vi "checkGST.vi"(0 "reference in":refnum<class "excelFile.lvclass">, 2 "TSR_details":T1={"Company/Institution:"="", "Address:"="", "Department:"="", "City:"="", "Post Code:"="", "Country:"="", "Contact:"="", "Ref:"="", "Issue description:"="", "Actions:"="", "TYPE:"="Repair", "Shipping:"=0, "Discount:"=0, "dataIN"=[], "Device type:"="microQuark", "Serial Number:"="", "PMC number:"="", "Labour Hours:"=0.0, "Service Location:"=FALSE, "start_hour"="", "end_hour"="", "o2_exp_date"="", "GST"=TRUE}, 5 "error in (no error)":errorcluster) -> (14 "reference out":refnum<class "excelFile.lvclass">, 19 "error out":errorcluster)   [LabVIEW 2016, in "excelFile.lvclass"]
uses:
  excelFile.lvclass
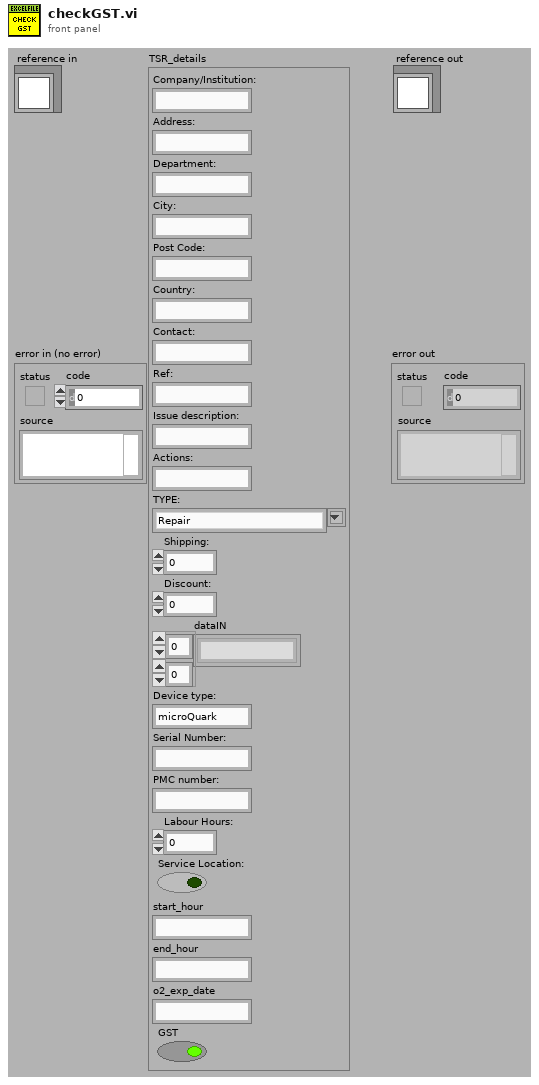
[diagram p1: front panel]
types:
  T1 = cluster{"Company/Institution:":string, "Address:":string, "Department:":string, "City:":string, "Post Code:":string, "Country:":string, "Contact:":string, "Ref:":string, "Issue description:":string, "Actions:":string, "TYPE:":string, "Shipping:":i32, "Discount:":i32, "dataIN":string[][], "Device type:":string, "Serial Number:":string, "PMC number:":string, "Labour Hours:":dbl, "Service Location:":bool, "start_hour":string, "end_hour":string, "o2_exp_date":string, "GST":bool}
  T2 = typedef "excelFile.lvclass/ObjectAttributesRef.ctl" = refnum<data-value>
  T3 = typedef "excelFile.lvclass/ObjectAttributes.ctl" = cluster{"MyAttribute":dbl, "path":string, "Refnum Excel":cluster{"Excel._Application":refnum<k7>, "Workbooks":refnum<k7>, "Open":refnum<k7>}, "data":string[][][], "save":bool, "fileType":T4, "rowsColor":u32[], "python_ref":refnum<class "python.lvclass">, "items_rows":i32[], "excel_range":i32[][], "TSR":cluster{"number":string, "TSR_path":path, "service_path":path, "email_to":string}, "excel_already_opened?":bool, "file_already_opened?":bool, "excel_protected_opened?":bool, "Refnum Cluster Worksheets":cluster{"Excel._Application":refnum<k7>, "Workbooks":refnum<k7>, "Open":refnum<k7>, "Worksheets":refnum<k7>, "Excel._Worksheet":refnum<k7>}, "#_rows_defective":i32, "#_rows_spare":i32}
  T4 = typedef "excelFile.lvclass/fileType.ctl" = enum16{"devices", "items", "partsTracking", "TSR"}
  T5 = cluster{"Excel._Application":refnum<k7>, "Workbooks":refnum<k7>, "Open":refnum<k7>, "Worksheets":refnum<k7>, "Excel._Worksheet":refnum<k7>}
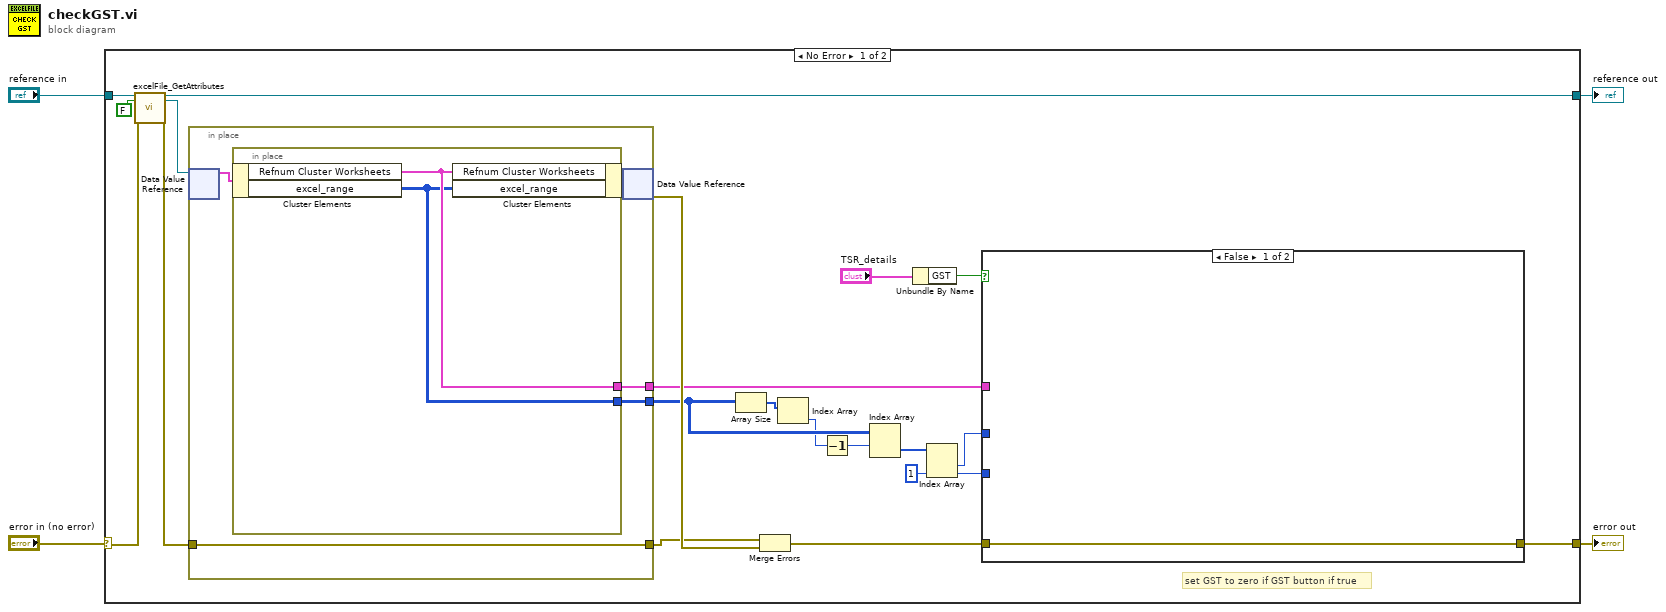
[diagram p0: block diagram]
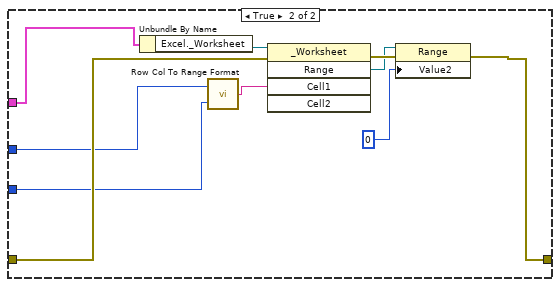
[diagram p2: hidden frame]
diagram:
  n1 = case shown="No Error" "error in (no error)" {
    selector: "error in (no error)" -> [w22 w45]
    tunnel: [w15 w45] -> w3
    tunnel: [w20 w44] -> w1
    tunnel: "reference in" -> [w24 w44]
    frame No Error {
      # "set GST to zero if GST button if true"
      n2 = call "excelFile_GetAttributes.vi"("reference in"=w24, "return data? (T)"=FALSE, "error in (no error)"=w22) -> ("reference out"=w20:refnum<class "excelFile.lvclass">, "attributes ref"=w19:T2, "error out"=w21:errorcluster)  [unwired: 13 in, 1 out]
      n3 = in-place {
        in-place-border: w21 -> [w39]
        in-place-border: [w39] -> w17
        in-place-border: [w38] -> w16
        in-place-border: [w37] -> w13
        n4 = in-place-dvr #1(w19) -> (w40:T3)  [unwired: 1 out]
        n5 = in-place {
          in-place-border: [w43] -> w38
          in-place-border: [w42] -> w37
          n6 = in-place-cluster #2(w40) -> ("Refnum Cluster Worksheets"=w43:T5, "excel_range"=w42:i32[][])
          n7 = in-place-cluster #2("Refnum Cluster Worksheets"=w43, "excel_range"=w42) -> (w41:T3)
        }
        n8 = in-place-dvr #1(w41) -> (w25:errorcluster)  [unwired: 1 out]
      }
      n9 = Array Size(array=w13) -> (size(s)=w12:i32[])
      n10 = Merge Errors(w17, w25) -> (w18:errorcluster)
      n11 = Index Array(array=w12) -> (element=w11:i32)  [unwired: 1 in]
      n12 = Decrement(x=w11) -> (x-1=w5:i32)
      n13 = Index Array(array=w13, index (row)=w5) -> (element=w10:i32[])  [unwired: 1 in]
      n14 = Unbundle By Name("TSR_details") -> ("GST"=w6:bool)
      n15 = Index Array(array=w10, index #2=1 ("index")) -> (element #1=w9:i32, element #2=w8:i32)  [unwired: 1 in]
      n16 = case shown="False" w6 {
        tunnel: w18 -> [w26 w36]
        tunnel: w16 -> [_ w35]
        tunnel: [w26 w34] -> w15
        tunnel: w9 -> [_ w29]
        tunnel: w8 -> [_ w28]
        frame False {
        }
        frame True {
          n17 = Unbundle By Name(w35) -> ("Excel._Worksheet"=w30:refnum<k7>)
          n18 = call <userlib>:"Row Col To Range Format.vi"("Column"=w28, "Row"=w29) -> ("Output String"=w33:string)
          n19 = invoke class="_Worksheet" method="Range"(reference=w30, error in=w36, "Cell1"=w33) -> (error out=w32:errorcluster, "Range"=w31:refnum<k7>)  [unwired: 2 in, 3 out]
          n20 = property class="Range"(reference=w31, error in=w32, "Value2"=0 ("index")) -> (error out=w34:errorcluster)  [unwired: 1 out]
        }
      }
    }
    frame Error {
    }
  }
  "error out" <- w3
  "reference out" <- w1
